vi "写入固件.vi"(8 "错误输入":errorcluster, 10 "selected path":path, 11 "MB session in":refnum<class "MB_Master.lvclass">) -> (0 "error out":errorcluster, 2 "结果字符串":string, 3 "MB session out":refnum<class "MB_Master.lvclass">)   [LabVIEW 2016, in "斯坦道总磷.lvlib"]
uses:
  <vilib>/Plasmionique/MB Master/MB_Master/MB_Master.lvclass
  <vilib>/NI/Progress Bar/Controls/Update Bar Actions.ctl
  <vilib>/Plasmionique/MB Master/MB_Master_Serial/MB_Master_Serial.lvclass
  C:/Program Files (x86)/National Instruments/LabVIEW 2016/vi.lib/Plasmionique/MB Master/MB_Master/MB_Master.lvclass
  <vilib>/Plasmionique/MB Master/MB Master.lvlib
  <vilib>/NI/Progress Bar/Progress Bar.lvlib
panel:
  out "error out 2":errorcluster caption="error out"
  in  "引用选择":enum16{"MB引用", "自建引用"}(ring)
  in  "VISA Resource":refnum<visa-resource-name>
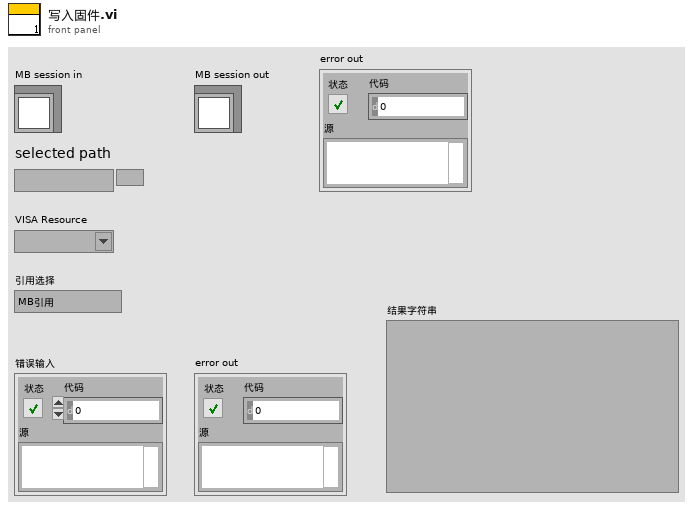
[diagram p1: front panel]
types:
  T1 = typedef "Progress Bar.lvlib/Update Bar Actions.ctl" = enum16{"Add To Existing", "Set to Value"}
  T2 = enum16{"open", "replace", "create", "open or create", "replace or create", "replace or create with confirmation"}
  T3 = enum16{"big-endian, network order", "native, host order", "little-endian"}
  T4 = cluster{"baud rate (bps)":u32, "stop bits":u16, "parity":u16, "flow control":u16, "timeout":u32, "retries":i32}
  T5 = typedef "SingleStepTestV3.lvlib/SingleStepTestV3.lvclass/仪器版本.ctl" = enum16{"V3.1版", "V4版", "V3版", "V4.2版"}
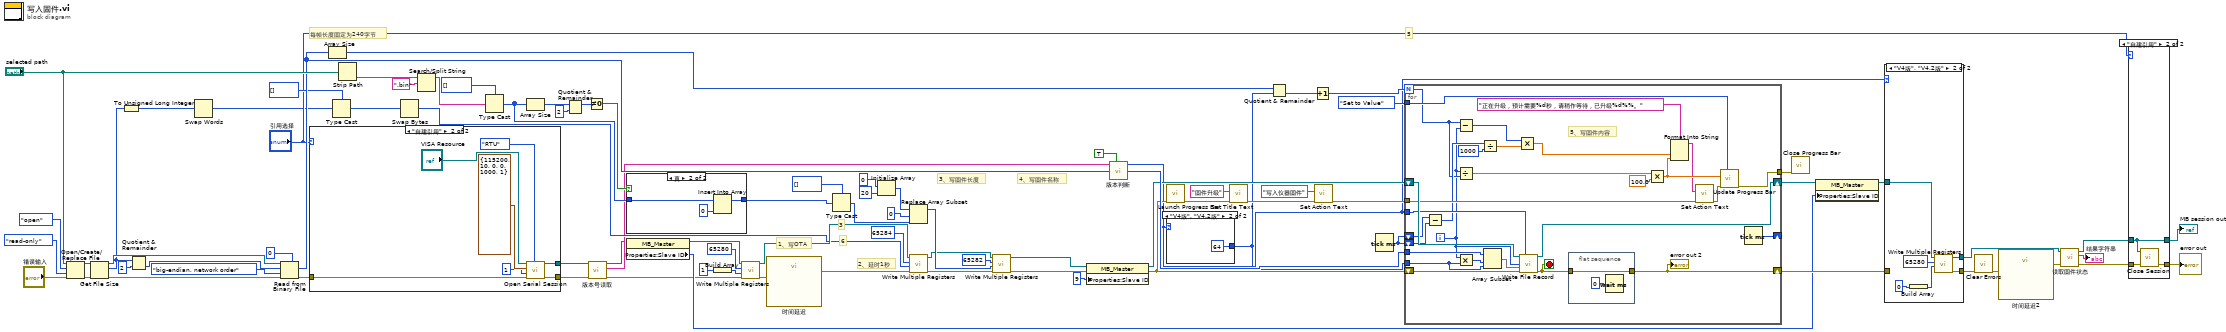
[diagram p0: block diagram]
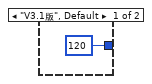
[diagram p2: hidden frame]
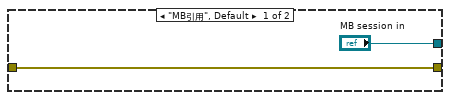
[diagram p6: hidden frame]
diagram:
  # "3"
  # "6"
  # "4、写固件名称"
  # "3、写固件长度"
  # "1、写OTA"
  # "5"
  # "每帧长度固定为240字节"
  # "2、延时1秒"
  n1 = Open/Create/Replace File(file path (use dialog)="selected path", error in="错误输入", operation (0:open)=T2."open" ("操作(0:open)"), access (0:read/write)=enum16{"read/write", "read-only", "write-only"}."read-only" ("权限(0:read/write)")) -> (refnum out=w77:refnum<file>, error out=w75:errorcluster)  [unwired: 2 in, 1 out]
  n2 = Get File Size(file=w77, error in=w75) -> (refnum out=w76:refnum<file>, size (in bytes)=w70:i64, 0:w74:errorcluster)
  n3 = To Unsigned Long Integer(number=w70) -> (unsigned 32bit integer=w51:u32)
  n4 = Quotient & Remainder(x=w70, y=i64 2) -> (floor(x/y)=w72:i64)  [unwired: 1 out]
  n5 = Swap Words(1:w51) -> (0:w50:u32)
  n6 = Read from Binary File(5:u16 0, 8:w74, 9:T3."big-endian, network order" ("字节顺序(0:big-endian, network order)"), 10:w72, 11:w76) -> (0:w78:errorcluster, 2:w71:u16[])  [unwired: 1 in, 2 out]
  n7 = case shown="\"自建引用\"" "引用选择" {
    tunnel: ["MB session in" w94] -> w5
    tunnel: w78 -> [w88 w93]
    tunnel: [w88 w92] -> w3
    frame "MB引用", Default {
    }
    frame "自建引用" {
      n8 = call <vilib>:"Open Serial Session.vi"("Mode (RTU)"=enum16{"RTU", "ASCII"}."RTU", "Error in"=w93, "Slave ID"=u8 1, "Serial Config"=T4 {"baud rate (bps)"=115200, "stop bits"=10, "parity"=0, "flow control"=0, "timeout"=1000, "retries"=1}, "VISA Resource"="VISA Resource") -> ("Error out"=w92:errorcluster, "MB_Serial session"=w94:refnum<class "MB_Master_Serial.lvclass">)  [unwired: 5 in]
    }
  }
  n9 = Array Size(array=w71) -> (size(s)=w69:i32)
  n10 = Type Cast(type=u16[] [], x=w50) -> (*(type *) &x=w65:u16[])
  n11 = Strip Path(path="selected path") -> (name=w79:string)  [unwired: 1 out]
  n12 = Swap Bytes(anything=w65) -> (byte swapped=w42:u16[])
  n13 = Search/Split String(string=w79, search string/char (-)=".bin" ("搜索字符串/字符(-)")) -> (substring before match=w60:string)  [unwired: 1 in, 2 out]
  n14 = Type Cast(type=u8[] [], x=w60) -> (*(type *) &x=w44:u8[])
  n15 = Array Size(array=w44) -> (size(s)=w48:i32)
  n16 = Quotient & Remainder(x=w48, y=2) -> (x-y*floor(x/y)=w46:i32)  [unwired: 1 out]
  n17 = Not Equal To 0?(x=w46) -> (x != 0?=w45:bool)
  n18 = call "版本号读取.vi"("Error in"=w3, "MB session in"=w5) -> ("error out"=w2:errorcluster, "固件版本号"=w9:string, "MB session out"=w4:refnum<class "MB_Master.lvclass">)  [unwired: 7 in]
  n19 = case shown="真" w45 {
    tunnel: w44 -> [w96 w99]
    tunnel: [w96 w98] -> w43
    frame False {
    }
    frame True {
      n20 = Insert Into Array(array=w99, new element=u8 0 ("新元素/子数组")) -> (w98:u8[])  [unwired: 1 in]
    }
  }
  n21 = property class="MB_Master"(reference=w4) -> (reference out=w20:refnum<class "MB_Master.lvclass">, "Properties:Slave ID"=w18:u8)  [unwired: 1 in, 1 out]
  n22 = Build Array(u16 1 ("value")) -> (w62:u16[])
  n23 = call <vilib>:"Write Multiple Registers.vi"("error in (no error)"=w2, "values"=w62, "starting address"=u16 65280, "MB session in"=w20) -> ("error out"=w67:errorcluster, "MB session out"=w57:refnum<class "MB_Master.lvclass">)  [unwired: 6 in]
  n24 = call "时间延迟"("error in (no error)"=w67) -> ("error out"=w58:errorcluster)  [unwired: 10 in]
  n25 = Type Cast(type=u16[] [], x=w43) -> (*(type *) &x=w26:u16[])
  n26 = Initialize Array(u16 0, 20 ("维数大小")) -> (w27:u16[])
  n27 = Replace Array Subset(array=w27, new element=w26, index=0 ("索引")) -> (w24:u16[])
  n28 = call <vilib>:"Write Multiple Registers.vi"("error in (no error)"=w58, "values"=w42, "starting address"=u16 65284, "MB session in"=w57) -> ("error out"=w7:errorcluster, "MB session out"=w8:refnum<class "MB_Master.lvclass">)  [unwired: 6 in]
  n29 = call <vilib>:"Write Multiple Registers.vi"("error in (no error)"=w7, "values"=w24, "starting address"=u16 65282, "MB session in"=w8) -> ("error out"=w52:errorcluster, "MB session out"=w55:refnum<class "MB_Master.lvclass">)  [unwired: 6 in]
  n30 = property class="MB_Master"(reference=w55, error in=w52, "Properties:Slave ID"=u8 9 ("Slave ID")) -> (reference out=w53:refnum<class "MB_Master.lvclass">, error out=w32:errorcluster)
  n31 = call "版本判断.vi"("Extern"=TRUE, "固件版本号"=w9) -> ("仪器版本"=w17:T5)  [unwired: 9 in]
  n32 = call <vilib>:"Launch Progress Bar.vi"("error in (no error)"=w32) -> ("error out"=w35:errorcluster)  [unwired: 9 in, 1 out]
  n33 = case shown="\"V4版\", \"V4.2版\"" w17 {
    tunnel: [120 ("y") 64 ("y")] -> w16
    frame "V3.1版", Default {
    }
    frame "V4版", "V4.2版" {
    }
  }
  n34 = call <vilib>:"Set Title Text.vi"("error in (no error)"=w35, "Installer Title"="固件升级") -> ("error out"=w34:errorcluster)  [unwired: 9 in]
  n35 = Quotient & Remainder(x=w69, y=w16) -> (floor(x/y)=w41:i32)  [unwired: 1 out]
  n36 = Increment(x=w41) -> (x+1=w56:i32)
  n37 = call <vilib>:"Set Action Text.vi"("error in (no error)"=w34, "Action Text"="写入仪器固件") -> ("error out"=w37:errorcluster)  [unwired: 9 in]
  n38 = Tick Count (ms)() -> (millisecond timer value=w1:u32)
  n39 = for {
    N: w56 -> [w109]
    shift-right: [w128] -> w23
    shift-left: w53 -> [w130]
    shift-right: [w116] -> w22
    shift-left: w32 -> [w129]
    tunnel: w71 -> [w126]
    tunnel: Update_Bar_Actions."Set to Value" ("Action") -> [w123]
    tunnel: [w122] -> w36
    tunnel: w37 -> [w114]
    tunnel: w17 -> [w113]
    tunnel: w16 -> [w112]
    shift-right: [w102] -> _
    shift-left: w1 -> [w104]
    shift-left: w1 -> [w103]
    i -> [w108]
    stop <- w117 stop-if-true
    # "5、写固件内容"
    n40 = Subtract(x=w104, y=w103) -> (x-y=w111:u32)
    n41 = Subtract(x=w109, y=w108) -> (x-y=w107:i32)
    n42 = Divide(x=w108, y=w109) -> (x/y=w119:dbl)
    n43 = Multiply(x=w108, y=w112) -> (x*y=w124:i32)
    n44 = Divide(x=w111, y=u32 1000) -> (x/y=w106:dbl)
    n45 = Array Subset(array=w126, index=w124, length=w112) -> (w125:u16[])
    n46 = Multiply(x=w107, y=w106) -> (x*y=w105:dbl)
    n47 = call "Write File Record.vi"("MB session in"=w130, "仪器版本"=w113, "Record Number"=w108, "values"=w125, "error in (no error)"=w129) -> ("MB session out"=w128:refnum<class "MB_Master.lvclass">, "error out"=w117:errorcluster)  [unwired: 9 in]
    n48 = flat-sequence {
      tunnel: w117 -> [w132]
      tunnel: [w132] -> w116
      frame #0 {
        n49 = Wait (ms)(milliseconds to wait=u32 0 ("等待时间（毫秒）")) -> ()  [unwired: 1 out]
      }
    }
    n50 = Multiply(x=w119, y=100.0) -> (x*y=w118:dbl)
    n51 = Format Into String(format string="正在升级，预计需要%d秒，请稍作等待，已升级%d%%。" ("格式字符串"), w105, w118) -> (resulting string=w115:string)  [unwired: 2 in, 1 out]
    n52 = call <vilib>:"Set Action Text.vi"("error in (no error)"=w114, "Action Text"=w115) -> ("error out"=w121:errorcluster)  [unwired: 9 in]
    n53 = call <vilib>:"Update Progress Bar.vi"("Action"=w123, "error in (no error)"=w121, "Value"=w118) -> ("error out"=w122:errorcluster)  [unwired: 8 in]
    n54 = Tick Count (ms)() -> (millisecond timer value=w102:u32)
    "error out 2" <- w116
  }
  n55 = call <vilib>:"Close Progress Bar.vi"("error in (no error)"=w36) -> ()  [unwired: 9 in, 2 out]
  n56 = property class="MB_Master"(reference=w23, "Properties:Slave ID"=w18) -> (reference out=w19:refnum<class "MB_Master.lvclass">)  [unwired: 1 in, 1 out]
  n57 = case shown="\"V4版\", \"V4.2版\"" w17 {
    tunnel: w19 -> [w133 w137]
    tunnel: [w133 w136] -> w14
    tunnel: w22 -> [w134 _]
    tunnel: [w134 w135] -> w21
    frame "V3.1版", Default {
    }
    frame "V4版", "V4.2版" {
      n58 = Build Array(0 ("value")) -> (w138:i32[])
      n59 = call <vilib>:"Write Multiple Registers.vi"("values"=w138, "starting address"=u16 65280, "MB session in"=w137) -> ("error out"=w135:errorcluster, "MB session out"=w136:refnum<class "MB_Master.lvclass">)  [unwired: 7 in]
    }
  }
  n60 = call <vilib>:"Clear Errors.vi"("error in (no error)"=w21) -> ("error out"=w40:errorcluster)  [unwired: 5 in, 1 out]
  n61 = call "时间延迟2"("error in (no error)"=w40) -> ("error out"=w15:errorcluster)  [unwired: 10 in]
  n62 = call "读取固件状态.vi"("错误输入"=w15, "MB session in"=w14) -> ("error out"=w12:errorcluster, "结果字符串"=→"结果字符串":string, "MB session out"=w13:refnum<class "MB_Master.lvclass">)  [unwired: 6 in, 1 out]
  n63 = case shown="\"自建引用\"" "引用选择" {
    tunnel: w13 -> [w141 w143]
    tunnel: w12 -> [w142 w145]
    tunnel: [w142 w144] -> w85
    tunnel: [w141 w143] -> w39
    frame "MB引用", Default {
    }
    frame "自建引用" {
      n64 = call-dynamic "Close Session.vi"("error in (no error)"=w145, "MB session in"=w143) -> ("error out"=w144:errorcluster)  [unwired: 9 in]
    }
  }
  "error out" <- w85
  "MB session out" <- w39
